vi "Example Simple.vi"() -> ()   [LabVIEW 2013]
uses:
  C:/tf/play/labview/Tinkerforge.dll
  Tinkerforge.dll
panel:
  out "temperature (°C)":sgl
  in  "uid":string="dHd"
  in  "port":i32=4223
  in  "host":string="localhost"
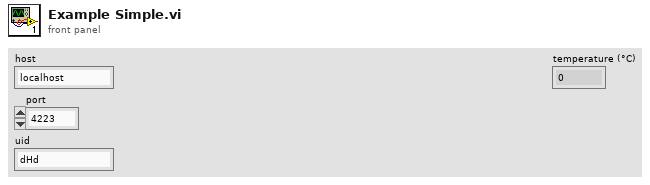
[diagram p1: front panel]
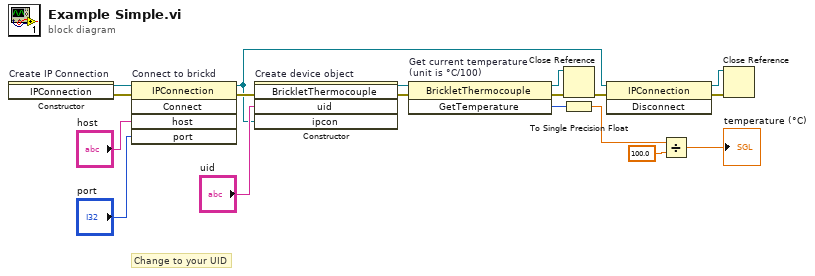
[diagram p0: block diagram]
diagram:
  # "Change to your UID"
  n1 = constructor on="Create IP Connection" class="IPConnection"() -> (reference out=w18:refnum<k24>, error out=w1:errorcluster)  [unwired: 3 in, 1 out]
  n2 = invoke on="Connect to brickd" class="IPConnection" method="Connect"(reference=w18, error in=w1, "host"="host", "port"="port") -> (reference out=w7:refnum<k24>, error out=w14:errorcluster)  [unwired: 1 in, 3 out]
  n3 = constructor on="Create device object" class="BrickletThermocouple"(error in=w14, "uid"="uid", "ipcon"=w7) -> (reference out=w12:refnum<k24>, error out=w13:errorcluster)  [unwired: 2 in, 3 out]
  n4 = invoke on="Get current temperature\n(unit is °C/100)" class="BrickletThermocouple" method="GetTemperature"(reference=w12, error in=w13) -> (reference out=w10:refnum<k24>, error out=w11:errorcluster, "GetTemperature"=w5:i32)  [unwired: 1 in]
  n5 = Close Reference(reference=w10, error in (no error)=w11) -> (error out=w9:errorcluster)
  n6 = To Single Precision Float(number=w5) -> (single precision float=w3:sgl)
  n7 = invoke class="IPConnection" method="Disconnect"(reference=w7, error in=w9) -> (reference out=w6:refnum<k24>, error out=w8:errorcluster)  [unwired: 1 in, 1 out]
  n8 = Divide(x=w3, y=sgl 100.0) -> (x/y=→"temperature (°C)":sgl)
  n9 = Close Reference(reference=w6, error in (no error)=w8) -> ()  [unwired: 1 out]
